vi "epxMAUpdate1bitword.vi"(6 "input valid":bool=TRUE, 8 "expFactor":i16=-8, 10 "update":fxp<+/-,22,2>, 11 "carryIn":fxp<+/-,22,2>) -> (0 "output valid":bool, 3 "carryOut":fxp<+/-,22,2>)   [LabVIEW 2016]
uses:
  <vilib>/rvi/FXPMathLib/FxpSub/XNode/nifxpmath_Sub.xnode
  <vilib>/rvi/FXPMathLib/FxpAdd/XNode/nifxpmath_Add.xnode
  <vilib>/rvi/FXPMathLib/sim/FxpSim.dll
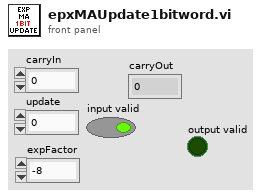
[diagram p1: front panel]
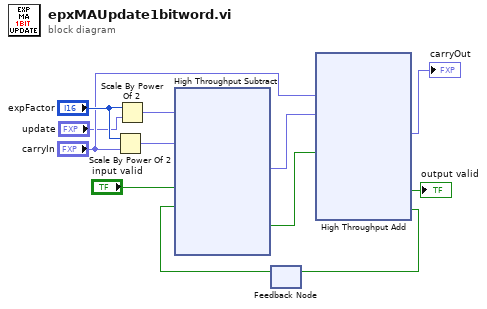
[diagram p0: block diagram]
diagram:
  n1 = Scale By Power Of 2(n="expFactor", x="carryIn") -> (x*2^n=w10:fxp<+/-,22,2>)
  n2 = Scale By Power Of 2(n="expFactor", x="update") -> (x*2^n=w11:fxp<+/-,22,2>)
  n3 = feedback #1() -> (w3:bool)  [unwired: 1 in]
  n4 = xnode "High Throughput Subtract"("x"=w11, "y"=w10, "input valid"="input valid", "ready for output (T)"=w3) -> ("x-y"=w8:fxp<+/-,22,2>, "output valid"=w5:bool)  [unwired: 1 out]
  n5 = xnode ("High Throughput Add")("x"="carryIn", "y"=w8, "input valid"=w5) -> ("x+y"=→"carryOut":fxp<+/-,22,2>, "output valid"=→"output valid":bool, "ready for input"=w4:bool)  [unwired: 1 in]
  n6 = feedback-in #1(w4) -> ()
